vi "get_mean_current.vi"(8 "error in (no error)":errorcluster, 10 "Channel":i8, 11 "TecellaClient in":refnum<class "TecellaClient.lvclass">) -> (0 "error out":errorcluster, 2 "Mean Current (nA)":dbl, 3 "TecellaClient out":refnum<class "TecellaClient.lvclass">)   [LabVIEW 2009, in "TecellaClient.lvclass"]
uses:
  TecellaClient.lvclass
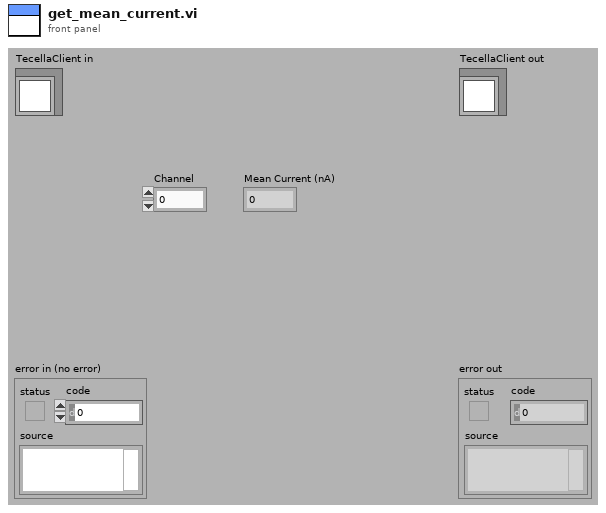
[diagram p1: front panel]
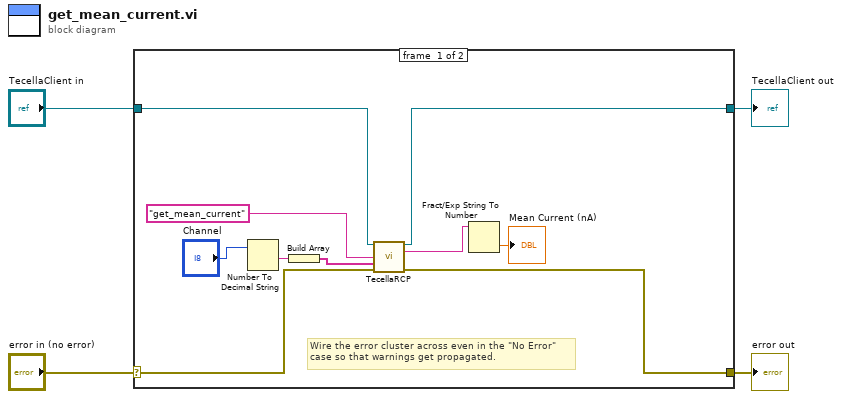
[diagram p0: block diagram]
diagram:
  n1 = case shown="No Error" "error in (no error)" {
    selector: "error in (no error)" -> [w9 w16]
    tunnel: [w8 w16] -> w3
    tunnel: [w7 w15] -> w1
    tunnel: "TecellaClient in" -> [w10 w15]
    frame #0 {
      # "Wire the error cluster across even in the \"No Error\"\ncase so that warnings get propagated."
      n2 = Number To Decimal String(number="Channel") -> (decimal integer string=w12:string)  [unwired: 1 in]
      n3 = Build Array(w12) -> (w13:string[])
      n4 = call-dynamic "TecellaRCP.vi"("TecellaClient in"=w10, "method"="get_mean_current", "Args"=w13, "error in (no error)"=w9) -> ("TecellaClient out"=w7:refnum<class "TecellaClient.lvclass">, "Data Returned"=w6:string, "error out"=w8:errorcluster)  [unwired: 9 in]
      n5 = Fract/Exp String To Number(string=w6) -> (number=→"Mean Current (nA)":dbl)  [unwired: 3 in, 1 out]
    }
    frame #1 {
    }
  }
  "error out" <- w3
  "TecellaClient out" <- w1
